vi "Drive.vi"(6 "Wheel DevRef":T1={"DeviceStatus"={"status"=FALSE, "code"=0, "source"=""}, "Type"=enum."PWM", "PWM"={"PWM Channel"=enum."Invalid", "DeadBand"={"Name"="", "maxPositivePwm"=0, "minPositivePwm"=0, "centerPwm"=0, "maxNegativePwm"=0, "minNegativePwm"=0, "angularRange"=0}}, "CAN"={"Device Number"=0, "SetOutput VI Ref"=variant(refnum<vi> refnum), "GetOutput VI Ref"=variant(refnum<vi> refnum), "Enable VI Ref"=variant(refnum<vi> refnum), "Disable VI Ref"=variant(refnum<vi> refnum), "Data"=variant}, "Invert"=FALSE}, 7 "Swerve DevRef":T1={"DeviceStatus"={"status"=FALSE, "code"=0, "source"=""}, "Type"=enum."PWM", "PWM"={"PWM Channel"=enum."PWM 1", "DeadBand"={"Name"="", "maxPositivePwm"=0, "minPositivePwm"=0, "centerPwm"=0, "maxNegativePwm"=0, "minNegativePwm"=0, "angularRange"=0}}, "CAN"={"Device Number"=0, "SetOutput VI Ref"=variant(enum8{"Percent VBus", "Current", "Speed", "Position", "Voltage"} enum."Percent VBus"), "GetOutput VI Ref"=variant(refnum<k1> refnum), "Enable VI Ref"=variant(dbl 12.0), "Disable VI Ref"=variant(enum8{"Percent VBus", "Speed", "Position", "Slave", "Unchanged / Invalid", "Voltage Compensation", "Current", "Motion Profile"} enum."Percent VBus"), "Data"=variant}, "Invert"=FALSE}, 8 "error in":errorcluster, 9 "Index":i32, 10 "Max Speed or 1":dbl, 11 "constants":cluster{"a":dbl, "b":dbl, "c":dbl, "d":dbl}) -> (0 "Reverse?":bool, 1 "Wheel Speed":dbl, 2 "Setpoint":dbl, 3 "Swerve Speed":dbl, 4 "error out":errorcluster)   [LabVIEW 2016]
uses:
  <vilib>/Rock Robotics/WPI/MotorControl/WPI_MotorControlDeviceRef.ctl
  <vilib>/Rock Robotics/WPI/MotorControl/WPI_MotorControlType.ctl
  <vilib>/Rock Robotics/SystemInterfaces/DIO/FPGA_DIOPWMChannel.ctl
  <vilib>/Rock Robotics/WPI/PWM/WPI_PWMDeadband.ctl
  <vilib>/ptbypt/NI_PtbyPt.lvlib
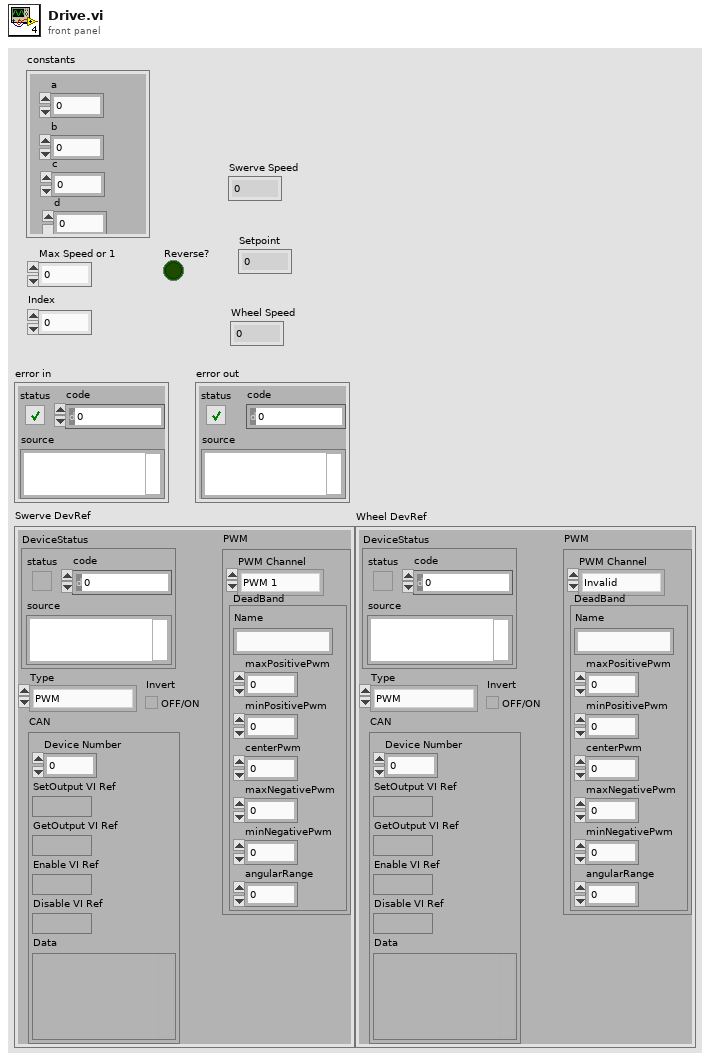
[diagram p1: front panel]
types:
  T1 = typedef "WPI_MotorControlDeviceRef.ctl" = cluster{"DeviceStatus":errorcluster, "Type":T2, "PWM":cluster{"PWM Channel":T3, "DeadBand":T4}, "CAN":cluster{"Device Number":u8, "SetOutput VI Ref":variant, "GetOutput VI Ref":variant, "Enable VI Ref":variant, "Disable VI Ref":variant, "Data":variant}, "Invert":bool}
  T2 = typedef "WPI_MotorControlType.ctl" = enum16{"PWM", "CAN"}
  T3 = typedef "FPGA_DIOPWMChannel.ctl" = enum8{"PWM 0", "PWM 1", "PWM 2", "PWM 3", "PWM 4", "PWM 5", "PWM 6", "PWM 7", "PWM 8", "PWM 9", "PWM MXP 0", "PWM MXP 1", "PWM MXP 2", "PWM MXP 3", "PWM MXP 4", "PWM MXP 5", "PWM MXP 6", "PWM MXP 7", "PWM MXP 8", "PWM MXP 9", "Invalid"}
  T4 = typedef "WPI_PWMDeadband.ctl" = cluster{"Name":string, "maxPositivePwm":i32, "minPositivePwm":i32, "centerPwm":i32, "maxNegativePwm":i32, "minNegativePwm":i32, "angularRange":u16}
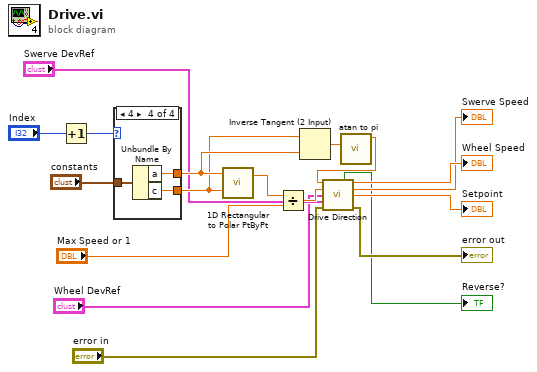
[diagram p0: block diagram]
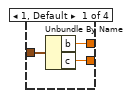
[diagram p2: hidden frame]
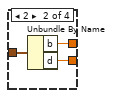
[diagram p3: hidden frame]
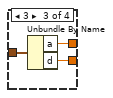
[diagram p4: hidden frame]
diagram:
  n1 = Increment(x="Index") -> (x+1=w16:i32)
  n2 = case shown="4" w16 {
    tunnel: "constants" -> [w21 w24 w27 w30]
    tunnel: [w20 w23 w26 w29] -> w12
    tunnel: [w19 w22 w25 w28] -> w11
    frame 1, Default {
      n3 = Unbundle By Name(w21) -> ("b"=w20:dbl, "c"=w19:dbl)
    }
    frame 2 {
      n4 = Unbundle By Name(w24) -> ("b"=w23:dbl, "d"=w22:dbl)
    }
    frame 3 {
      n5 = Unbundle By Name(w27) -> ("a"=w26:dbl, "d"=w25:dbl)
    }
    frame 4 {
      n6 = Unbundle By Name(w30) -> ("a"=w29:dbl, "c"=w28:dbl)
    }
  }
  n7 = call <vilib>:"1D Rectangular to Polar PtByPt.vi"("y"=w11, "x"=w12) -> ("magnitude"=w15:dbl)  [unwired: 1 out]
  n8 = Divide(x=w15, y="Max Speed or 1") -> (x/y=w13:dbl)
  n9 = Inverse Tangent (2 Input)(1:w12, 2:w11) -> (0:w10:dbl)
  n10 = call "atan to pi.vi"("atan2 result"=w10) -> ("Scaled"=w9:dbl)  [unwired: 10 in]
  n11 = call "Drive Direction.vi"("Desired direction (radians)"=w9, "Wheel Power"=w13, "Wheel DevRef"="Wheel DevRef", "Swerve DevRef"="Swerve DevRef", "error in"="error in") -> ("Reverse?"=→"Reverse?":bool, "Wheel Speed"=→"Wheel Speed":dbl, "Swerve Speed"=→"Swerve Speed":dbl, "Setpoint"=→"Setpoint":dbl, "error out"=→"error out":errorcluster)  [unwired: 6 in]
